vi "XY Graph Compute (f,g)(X,Y) Arrays.vi"(8 "Error In":errorcluster, 9 "Formulas":string[](array[string]), 10 "Y Array":dbl[](array[numeric]), 11 "X Array":dbl[](array[numeric])) -> (0 "Error Out":errorcluster, 1 "Formula String":string, 2 "g(X,Y) Array":dbl[](array[numeric]), 3 "f(X,Y) Array":dbl[](array[numeric]))   [LabVIEW 2021, in "XY Graph Add-Ons.lvlib"]
uses:
  XY Graph Add-Ons.lvlib
  <vilib>/gmath/NI_Gmath.lvlib
  Strings/Strings.lvlib
  Utilities/Utilities.lvlib
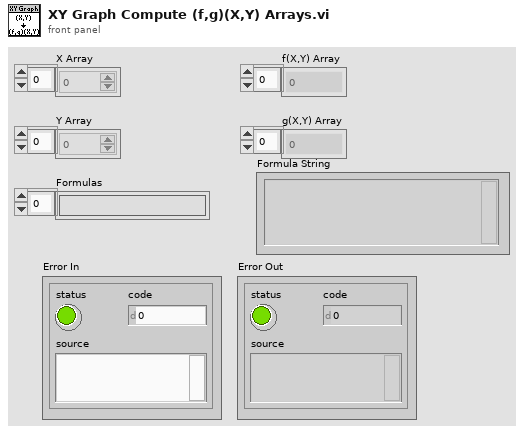
[diagram p1: front panel]
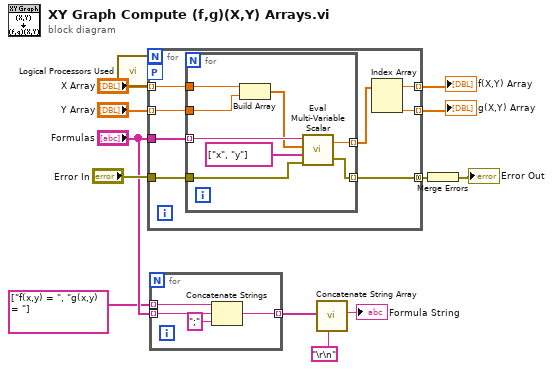
[diagram p0: block diagram]
diagram:
  n1 = call "Logical Processors Used.vi"() -> ("# Logical Processor Used"=w1:i32)  [unwired: 6 in]
  n2 = for {
    tunnel: "X Array" -> [w20] mode=indexing
    tunnel: "Y Array" -> [w19] mode=indexing
    tunnel: [w15] -> w12 mode=indexing
    tunnel: [w14] -> w13 mode=indexing
    tunnel: "Formulas" -> [w21]
    tunnel: "Error In" -> [w18]
    workers-P: w1 -> [_]
    tunnel: [w17] -> w8 mode=concatenating
    n3 = for {
      tunnel: w21 -> [w29] mode=indexing
      tunnel: w20 -> [w27]
      tunnel: w19 -> [w26]
      tunnel: w18 -> [w24]
      tunnel: [w23] -> w17 mode=indexing
      tunnel: [w22] -> w16 mode=indexing
      n4 = Build Array(w27, w26) -> (w25:dbl[])
      n5 = call <vilib>:"Eval Multi-Variable Scalar.vi"("error in (no error)"=w24, "Variables"=string[] ["x", "y"], "X Values"=w25, "formula"=w29) -> ("error out"=w23:errorcluster, "y value"=w22:dbl)
    }
    n6 = Index Array(array=w16) -> (element #1=w15:dbl, element #2=w14:dbl)  [unwired: 2 in]
  }
  "g(X,Y) Array" <- w13
  "f(X,Y) Array" <- w12
  n7 = for {
    tunnel: "Formulas" -> [w32] mode=indexing
    tunnel: string[] ["f(x,y) = ", "g(x,y) = "] -> [w33] mode=indexing
    tunnel: [w30] -> w4 mode=indexing
    n8 = Concatenate Strings(w33, w32, ";" ("string")) -> (w30:string)
  }
  n9 = call "Concatenate String Array.vi"("Separator (TAB)"="\r\n", "String Array"=w4) -> ("Formatted String"=→"Formula String":string)  [unwired: 9 in]
  n10 = Merge Errors(w8) -> (→"Error Out":errorcluster)
